vi "Escritura_DB_log.vi"(3 "HMI Class 3.lvclass 2":refnum<class "HMI Class 3.lvclass">) -> (11 "HMI Class 3.lvclass":refnum<class "HMI Class 3.lvclass">)   [LabVIEW 2019, in "HMI Class 3.lvclass"]
uses:
  HMI Class 3.lvclass
  HMI Class 3.lvclass/HMI Class 3.ctl
  <vilib>/addons/database/Connection.llb/DB Tools Open Connec (Path).vi
  <vilib>/addons/database/NI_Database_API.lvlib
panel:
  out "error out":errorcluster
  in  "error in (no error)":errorcluster
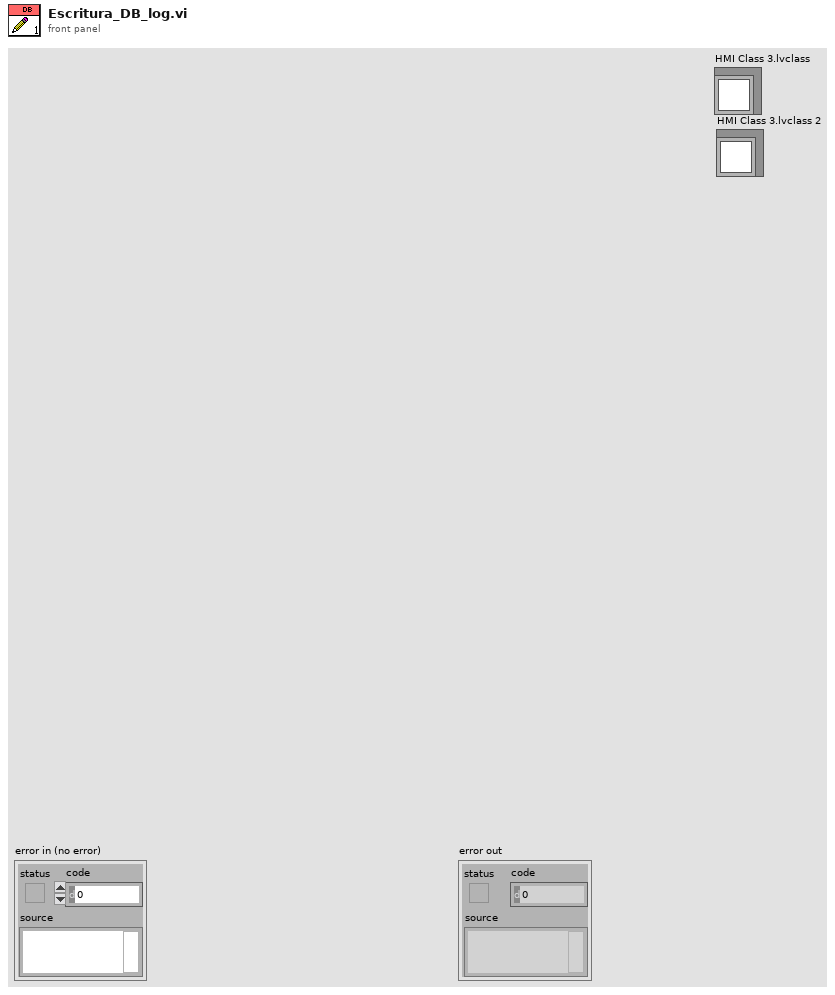
[diagram p1: front panel]
types:
  T1 = cluster{"MODELO":string, "JOB":i8, "LOTE":i8, "FECHA Y HORA":i8, "TENSION MEDIDA":i8, "GAP MEDIDA":i8, "TRIP GAP OK":i8}
  T2 = typedef "NI_Database_API.lvlib/Conn ObjectReference.ctl" = refnum<k1>
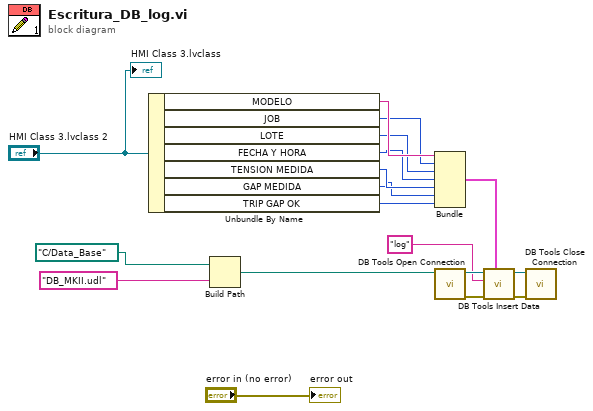
[diagram p0: block diagram]
diagram:
  n1 = Unbundle By Name("HMI Class 3.lvclass 2") -> ("MODELO"=w7:string, "JOB"=w6:i8, "LOTE"=w5:i8, "FECHA Y HORA"=w4:i8, "TENSION MEDIDA"=w3:i8, "GAP MEDIDA"=w2:i8, "TRIP GAP OK"=w1:i8)
  n2 = Build Path(base path=path "C:/Data_Base", name or relative path="DB_MKII.udl") -> (appended path=w17:path)
  n3 = Bundle("MODELO"=w7, "JOB"=w6, "LOTE"=w5, "FECHA Y HORA"=w4, "TENSION MEDIDA"=w3, "GAP MEDIDA"=w2, "TRIP GAP OK"=w1) -> (w12:T1)  [unwired: 1 in]
  n4 = call-poly <vilib>:"DB Tools Open Connection.vi"("connection information"=w17) -> ("error out"=w14:errorcluster, "connection reference"=w15:T2)  [unwired: 7 in]
  n5 = call <vilib>:"DB Tools Insert Data.vi"("data"=w12, "error in (no error)"=w14, "table"="log", "connection reference"=w15) -> ("error out"=w10:errorcluster, "connection reference out"=w11:T2)  [unwired: 6 in]
  n6 = call <vilib>:"DB Tools Close Connection.vi"("error in (no error)"=w10, "connection reference"=w11) -> ()  [unwired: 5 in, 1 out]
  "HMI Class 3.lvclass" <- "HMI Class 3.lvclass 2"
  "error out" <- "error in (no error)"
